vi "Number of lines in string.vi"(11 "Input string":string) -> (2 "Input string length":i32, 3 "Number of LF matches":i32, 5 "LF found?":bool)   [LabVIEW 2017]
uses:
  <vilib>/regexp/Match Regular Expression.xnode
panel:
  # "cmd.exe                    17160 Console                 0      3,196 K Running         GS66-BAMXP2\\shutters"
  # "Old programming/obsolete? (While loop at the bottom)"
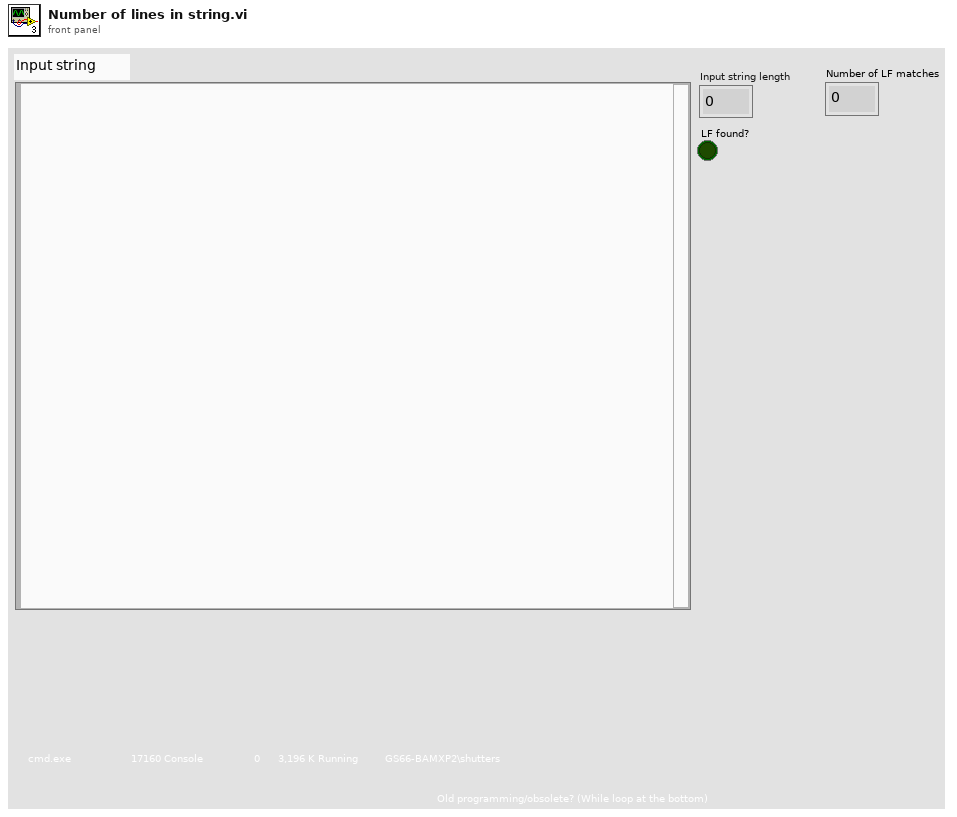
[diagram p1: front panel]
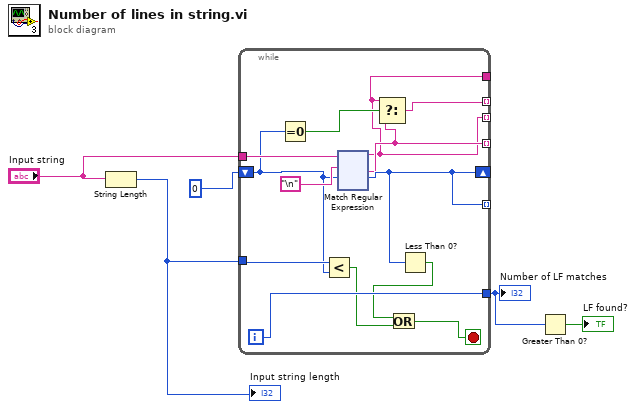
[diagram p0: block diagram]
diagram:
  n1 = String Length(string="Input string") -> (length=w4:i32)
  "Input string length" <- w4
  n2 = while {
    tunnel: "Input string" -> [w18]
    shift-right: [w15] -> _
    shift-left: 0 ("offset past token") -> [w7]
    tunnel: [w14] -> _ mode=indexing
    tunnel: [w11] -> _ mode=indexing
    tunnel: [w16] -> w1
    tunnel: [w15] -> _ mode=indexing
    tunnel: [w12] -> _ mode=indexing
    tunnel: [w11] -> _
    tunnel: w4 -> [w8]
    i -> [w16]
    stop <- w10 stop-if-true
    n3 = Equal To 0?(x=w7) -> (x = 0?=w13:bool)
    n4 = Less?(x=w8, y=w7) -> (x < y?=w6:bool)
    n5 = xnode "Match Regular Expression"("input string"=w18, "regular expression"="\n", "offset (0)"=w7) -> ("before match"=w11:string, "after match"=w14:string, "offset past match"=w15:i32)  [unwired: 3 in, 2 out]
    n6 = Select(t=w11, s=w13, f=w14) -> (s? t:f=w12:string)
    n7 = Less Than 0?(x=w15) -> (x < 0?=w9:bool)
    n8 = Or(x=w9, y=w6) -> (x .or. y?=w10:bool)
  }
  "Number of LF matches" <- w1
  n9 = Greater Than 0?(x=w1) -> (x > 0?=→"LF found?":bool)
